vi "Update application.vi"(8 "Error In":errorcluster) -> (0 "Error Out":errorcluster)   [LabVIEW 2017]
panel:
  out "Firefly iii App Container ID":string
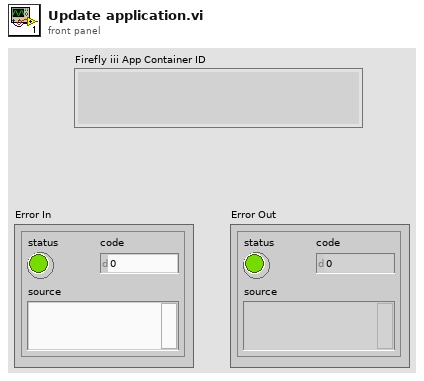
[diagram p1: front panel]
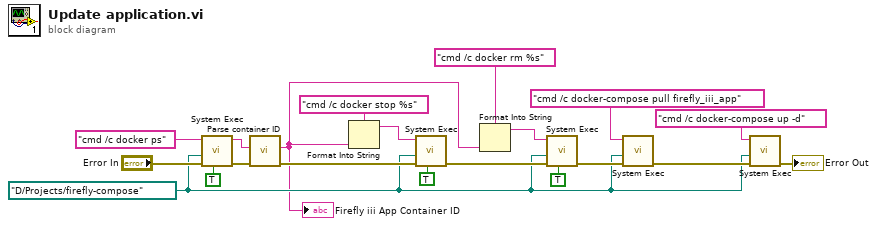
[diagram p0: block diagram]
diagram:
  w2 = path "D:/Projects/firefly-compose" ("working directory")
  n1 = call <vilib>:"System Exec.vi"("run minimized? (F)"=TRUE, "error in (no error)"="Error In", "working directory"=w2, "command line"="cmd /c docker ps") -> ("error out"=w18:errorcluster, "standard output"=w19:string)  [unwired: 4 in, 2 out]
  n2 = call "Parse container ID.vi"("Error In"=w18, "\"cmd /c docker ps\" output"=w19) -> ("Error Out"=w14:errorcluster, "Firefly iii App Container ID"=w1:string)  [unwired: 8 in]
  "Firefly iii App Container ID" <- w1
  n3 = Format Into String(format string="cmd /c docker stop %s" ("command line"), w1) -> (resulting string=w15:string)  [unwired: 2 in, 1 out]
  n4 = call <vilib>:"System Exec.vi"("run minimized? (F)"=TRUE, "error in (no error)"=w14, "working directory"=w2, "command line"=w15) -> ("error out"=w9:errorcluster)  [unwired: 4 in, 3 out]
  n5 = Format Into String(format string="cmd /c docker rm %s" ("command line"), w1) -> (resulting string=w7:string)  [unwired: 2 in, 1 out]
  n6 = call <vilib>:"System Exec.vi"("run minimized? (F)"=TRUE, "error in (no error)"=w9, "working directory"=w2, "command line"=w7) -> ("error out"=w5:errorcluster)  [unwired: 4 in, 3 out]
  n7 = call <vilib>:"System Exec.vi"("error in (no error)"=w5, "working directory"=w2, "command line"="cmd /c docker-compose pull firefly_iii_app") -> ("error out"=w4:errorcluster)  [unwired: 5 in, 3 out]
  n8 = call <vilib>:"System Exec.vi"("error in (no error)"=w4, "working directory"=w2, "command line"="cmd /c docker-compose up -d") -> ("error out"=→"Error Out":errorcluster)  [unwired: 5 in, 3 out]
